vi "Cmd Packet.vi"(2 "Command Byte":i32, 3 "Parameter Byte":u32) -> (0 "Command Packet Byte String":string, 1 "Command Packet Byte Array":u32[](array[numeric]))   [LabVIEW 2021]
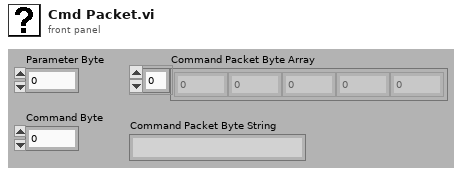
[diagram p1: front panel]
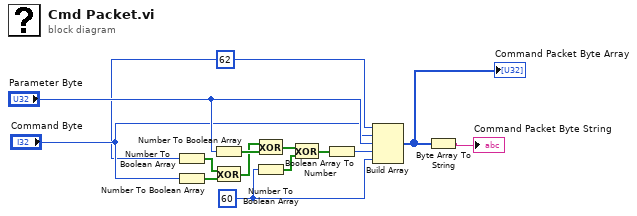
[diagram p0: block diagram]
diagram:
  w12 = 60 ("data in")
  w9 = 62 ("data in")
  n1 = Number To Boolean Array(number=w9) -> (Boolean array=w2:bool[])
  n2 = Number To Boolean Array(number="Command Byte") -> (Boolean array=w3:bool[])
  n3 = Number To Boolean Array(number="Parameter Byte") -> (Boolean array=w5:bool[])
  n4 = Exclusive Or(1:w3, 2:w2) -> (0:w4:bool[])
  n5 = Exclusive Or(1:w5, 2:w4) -> (0:w6:bool[])
  n6 = Number To Boolean Array(number=w12) -> (Boolean array=w7:bool[])
  n7 = Exclusive Or(1:w7, 2:w6) -> (0:w8:bool[])
  n8 = Boolean Array To Number(Boolean array=w8) -> (number=w11:u32)
  n9 = Build Array(w9, "Command Byte", "Parameter Byte", w11, w12) -> (w1:u32[])
  "Command Packet Byte Array" <- w1
  n10 = Byte Array To String(unsigned byte array=w1) -> (string=→"Command Packet Byte String":string)
